vi "Pockels Cal-Process window.vi"(8 "error in (no error)":errorcluster) -> (1 "Cancelled (Left button pressed)":bool, 3 "Timed out or errored out":bool)   [LabVIEW 2017]
doc: "Use this template to create a dialog box with event handling."
uses:
  AOL Z/Typedefs/Pockels cal process refs.ctl
  <vilib>/Utility/miscctls.llb/LVPointTypeDef.ctl
  Globals/gl_Calibration globals.vi
  Global Variables/General Globals.vi
panel:
  out "error out":errorcluster
  out "Measured Power ind":dbl caption="Measured Power (mW)" min=0.0 max=10000.0 step=1.0 format="%.1f"
  out "Abort objective":bool
  out "Pockels Cal table":string[][](array[string])
  in  "Measured Power ctrl":dbl caption="Enter Measured Power (mW)" min=0.0 max=10000.0 step=1.0 format="%#_6f"
  out "Pockels cal progress bar":u8(slide) scale=0.0..100.0
  out "Next (ind)":bool
  out "Cancelled/Aborted":bool
  out "Exit":bool
  out "Abort (ind)":bool
  out "Display message":string
  in  "Cancel":bool
  in  "Next":bool
  in  "Message string":string
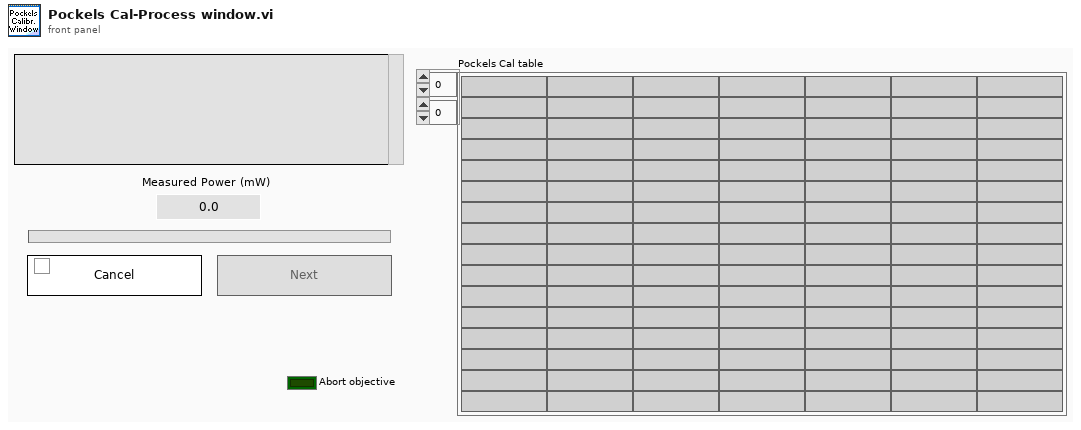
[diagram p1: front panel]
types:
  T1 = typedef "Pockels cal process refs.ctl" = cluster{"This VI":refnum<vi>, "Abort (ind)":refnum<vi>, "Next (ind)":refnum<vi>, "Cancel":refnum<vi>, "Next":refnum<vi>, "Message":refnum<vi>, "Measured Power ctrl":refnum<vi>, "Measured Power ind":refnum<vi>, "Pockels cal progress bar":refnum<vi>, "Abort this objective":refnum<vi>}
  T2 = typedef "LVPointTypeDef.ctl" = cluster{"Horizontal":i16, "Vertical":i16}
  T3 = typedef "Cal mode.ctl" = enum16{"Automatic", "Interactive"}
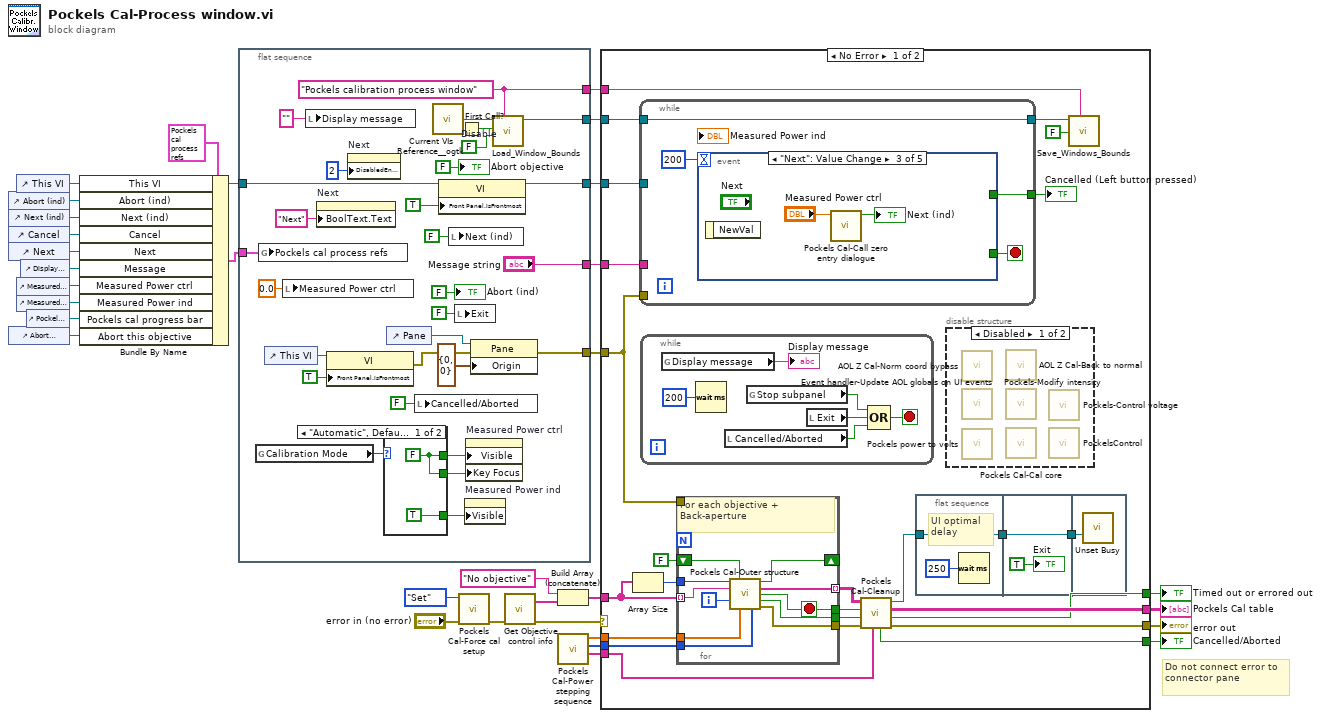
[diagram p0: block diagram]
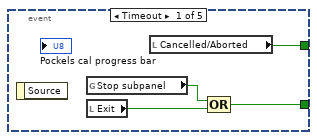
[diagram p3: hidden frame]
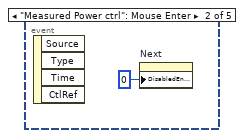
[diagram p4: hidden frame]
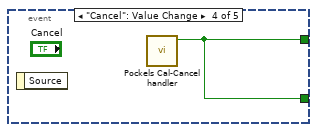
[diagram p5: hidden frame]
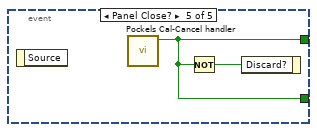
[diagram p6: hidden frame]
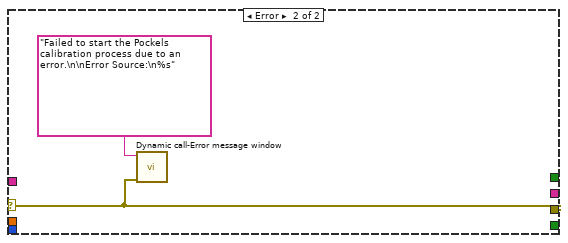
[diagram p7: hidden frame]
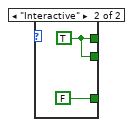
[diagram p8: hidden frame]
diagram:
  # "Do not connect error to connector pane"
  n1 = control-ref of="Abort (ind)"() -> (w26:refnum<vi>)
  n2 = control-ref of="Next (ind)"() -> (w25:refnum<vi>)
  n3 = control-ref of="Cancel"() -> (w24:refnum<vi>)
  n4 = control-ref of="Next"() -> (w23:refnum<vi>)
  n5 = control-ref of="Abort objective"() -> (w4:refnum<vi>)
  n6 = control-ref of="This VI"() -> (w22:refnum<vi>)
  n7 = control-ref of="Measured Power ctrl"() -> (w15:refnum<vi>)
  n8 = control-ref of="Measured Power ind"() -> (w1:refnum<vi>)
  n9 = control-ref of="Display message"() -> (w21:refnum<vi>)
  n10 = control-ref of="Pockels cal progress bar"() -> (w5:refnum<vi>)
  n11 = Bundle By Name(cluster=T1 {"This VI"=refnum, "Abort (ind)"=refnum, "Next (ind)"=refnum, "Cancel"=refnum, "Next"=refnum, "Message"=refnum, "Measured Power ctrl"=refnum, "Measured Power ind"=refnum, "Pockels cal progress bar"=refnum, "Abort this objective"=refnum} ("AOL Z cal wizard refs"), "This VI"=w22, "Abort (ind)"=w26, "Next (ind)"=w25, "Cancel"=w24, "Next"=w23, "Message"=w21, "Measured Power ctrl"=w15, "Measured Power ind"=w1, "Pockels cal progress bar"=w5, "Abort this objective"=w4) -> (w3:T1)
  n12 = flat-sequence {
    tunnel: ["Message string"] -> w31
    tunnel: [w58] -> w30
    tunnel: [w56] -> w27
    tunnel: [w51] -> w29
    tunnel: [w50] -> w28
    tunnel: w3 -> [w34]
    tunnel: w22 -> [w40]
    frame #0 {
      w52 = FALSE  # Disable
      w51 = "Pockels calibration process window" ("Window Name (i.e. Key)")
      n13 = global read "gl_Calibration globals.vi" "Calibration Mode"() -> (w33:T3)
      n14 = global write "gl_Calibration globals.vi" "Pockels cal process refs"(w34) -> ()
      n15 = control-ref of="This VI"() -> (w42:refnum<vi>)
      n16 = local write "Measured Power ctrl"(0.0 ("Measured Power")) -> ()
      n17 = local write "Display message"("" ("Status")) -> ()
      n18 = property on="Next" class="Bool"("BoolText.Text"="Next" ("Boolean Text.Text")) -> ()  [unwired: 2 in, 2 out]
      n19 = property on="Property Node" class="VI"(reference=w42, "Front Panel.IsFrontmost"=TRUE ("Front Panel Window:Is Frontmost")) -> (error out=w41:errorcluster)  [unwired: 1 in, 1 out]
      n20 = property on="Next" class="Bool"("DisabledEnum"=2) -> ()  [unwired: 2 in, 2 out]
      n21 = case shown="\"Automatic\", Default" w33 {
        tunnel: [w61 w63] -> w39
        tunnel: [w61 w63] -> w36
        tunnel: [TRUE FALSE] -> w32
        frame "Automatic", Default {
          w61 = FALSE
        }
        frame "Interactive" {
          w63 = TRUE
        }
      }
      n22 = control-ref of="Pane"() -> (w55:refnum<vi>)
      n23 = local write "Cancelled/Aborted"(FALSE ("Completed")) -> ()
      n24 = call <userlib>:"Current VIs Reference__ogtk.vi"() -> ("Current VI's reference"=w54:refnum<vi>)  [unwired: 5 in]
      n25 = property on="Property Node" class="VI"(reference=w40, "Front Panel.IsFrontmost"=TRUE ("Front Panel Window:Is Frontmost")) -> (reference out=w58:refnum<vi>)  [unwired: 1 in, 1 out]
      n26 = local write "Next (ind)"(FALSE ("Next (ind)")) -> ()
      n27 = local write "Exit"(FALSE ("Finished")) -> ()
      n28 = First Call?() -> (First Call?: T/F=w53:bool)
      n29 = property on="Measured Power ind" class="DigNum (strict)"("Visible"=w32) -> ()  [unwired: 2 in, 2 out]
      n30 = property on="Measured Power ctrl" class="DigNum (strict)"("Visible"=w39, "Key Focus"=w36) -> ()  [unwired: 2 in, 2 out]
      n31 = property class="Pane"(reference=w55, error in=w41, "Origin"=T2 {"Horizontal"=0, "Vertical"=0}) -> (error out=w56:errorcluster)  [unwired: 1 out]
      n32 = call "Load_Window_Bounds.vi"("Window Name (i.e. Key)"=w51, "Disable"=w52, "First Call"=w53, "Window VI's Ref"=w54) -> ("reference out"=w50:refnum<vi>)  [unwired: 4 in, 3 out]
      "Abort (ind)" <- FALSE ("Cancel ind")
      "Abort objective" <- FALSE ("Cancel ind")
    }
  }
  n33 = call "Pockels Cal-Force cal setup.vi"("error in (no error)"="error in (no error)", "Function"=enum16{"Set", "Recover"}."Set") -> ("error out"=w9:errorcluster)  [unwired: 9 in]
  n34 = call "Get Objective control info.vi"("error in (no error)"=w9) -> ("error out"=w18:errorcluster, "Objective values/strings"=w13:string[])  [unwired: 6 in, 3 out]
  n35 = Build Array (concatenate)("No objective" ("Value"), w13) -> (w12:string[])
  n36 = call "Pockels Cal-Power stepping sequence.vi"() -> ("Pockels calibration voltage steps sequence (strings)"=w17:string[], "Voltage %"=w14:u16[], "Pockels calibration voltage steps sequence"=w16:dbl[])  [unwired: 8 in, 1 out]
  n37 = case shown="No Error" w18 {
    selector: w18 -> [_ w126]
    tunnel: w31 -> [w89 _]
    tunnel: w30 -> [w88 _]
    tunnel: w29 -> [w87 _]
    tunnel: w28 -> [w85 _]
    tunnel: w27 -> [w82 _]
    tunnel: [w81 w126] -> w19
    tunnel: w12 -> [w76 _]
    tunnel: w17 -> [w69 _]
    tunnel: w16 -> [w79 _]
    tunnel: w14 -> [w78 _]
    tunnel: [w73 _] -> w7
    tunnel: [w72 _] -> w6
    tunnel: [w65 _] -> w2
    frame No Error {
      n38 = Array Size(array=w76) -> (size(s)=w77:i32)
      n39 = while {
        tunnel: w89 -> [_]
        tunnel: w82 -> [_]
        tunnel: w88 -> [_]
        tunnel: [w102] -> w74
        tunnel: w85 -> [w101]
        tunnel: [w101] -> w84
        stop <- w104 stop-if-true
        n40 = event shown="[2] \"Next\": Value Change" {
          selector: _ -> [_ _ _ _ _]
          dyn-events: _ -> [_ _ _ _ _]
          timeout: 200 -> [_ _ _ _ _]
          tunnel: [w107 _ _ w112 w114] -> w104
          tunnel: [w105 _ _ w112 w114] -> w102
          event Timeout {
            n41 = event-data() -> ()  [unwired: 1 in, 1 out]
            n42 = global read "General Globals.vi" "Stop subpanel"() -> (w106:bool)
            n43 = local read "Exit"() -> (w108:bool)
            n44 = local read "Cancelled/Aborted"() -> (w105:bool)
            n45 = Compound Arithmetic op=OR(w106, w108) -> (w107:bool)
          }
          event "Measured Power ctrl": Mouse Enter {
            n46 = event-data() -> ()  [unwired: 1 in, 4 out]
            n47 = property on="Next" class="Bool"("DisabledEnum"=0) -> ()  [unwired: 2 in, 2 out]
          }
          event "Next": Value Change {
            n48 = event-data() -> ()  [unwired: 1 in, 1 out]
            n49 = call "Pockels Cal-Call zero entry dialogue.vi"("Measured Power"="Measured Power ctrl") -> ("Next (ind)"=→"Next (ind)":bool)  [unwired: 10 in]
          }
          event "Cancel": Value Change {
            n50 = event-data() -> ()  [unwired: 1 in, 1 out]
            n51 = call "Pockels Cal-Cancel handler.vi"() -> ("Stop?"=w112:bool)  [unwired: 11 in]
          }
          event Panel Close? {
            n52 = event-data() -> ()  [unwired: 1 in, 1 out]
            n53 = call "Pockels Cal-Cancel handler.vi"() -> ("Stop?"=w114:bool)  [unwired: 11 in]
            n54 = Not(x=w114) -> (.not. x?=w113:bool)
            n55 = event-data("Discard?"=w113) -> ()  [unwired: 1 in, 1 out]
          }
        }
      }
      "Cancelled (Left button pressed)" <- w74
      n56 = while {
        stop <- w98 stop-if-true
        n57 = global read "gl_Calibration globals.vi" "Display message"() -> (→"Display message":string)
        n58 = Wait (ms)(milliseconds to wait=u32 200) -> ()  [unwired: 1 out]
        n59 = local read "Cancelled/Aborted"() -> (w95:bool)
        n60 = global read "General Globals.vi" "Stop subpanel"() -> (w100:bool)
        n61 = local read "Exit"() -> (w99:bool)
        n62 = Compound Arithmetic op=OR(w100, w99, w95) -> (w98:bool)
      }
      n63 = for {
        tunnel: [w125] -> w83 mode=indexing
        tunnel: [w115] -> w67
        tunnel: w82 -> [_]
        tunnel: [w116] -> w68
        tunnel: w77 -> [w124]
        tunnel: [w123] -> w80
        tunnel: w76 -> [w118] mode=indexing
        tunnel: w79 -> [w122]
        tunnel: w78 -> [w121]
        shift-right: [w120] -> _
        shift-left: FALSE -> [w119]
        i -> [w117]
        stop <- w115 stop-if-true
        # "For each objective + \nBack-aperture"
        n64 = call "Pockels Cal-Outer structure.vi"("Number of objectives + 1"=w124, "Skip cal for all remaining objectives?"=w119, "Objective's name"=w118, "Parent FOR loop's index"=w117, "Pockels calibration voltage steps sequence"=w122, "Voltage %"=w121) -> ("Skip cal for all remaining objectives"=w120:bool, "Results array"=w125:string[], "Cancel & Exit"=w115:bool, "Timed out or errored out"=w116:bool, "error out"=w123:errorcluster)  [unwired: 5 in]
      }
      n65 = call "Pockels Cal-Cleanup.vi"("Pockels calibration voltage steps sequence (strings)"=w69, "error in (no error)"=w80, "Timed out or error"=w68, "Cancelled/Aborted"=w67, "Calibration data (all objectives even if blank)"=w83) -> ("error out"=w81:errorcluster, "Timed out or errored out"=w72:bool, "Formatted cal table (inc. header)"=w73:string[][], "VI out"=w70:refnum<vi>, "Cancelled/Aborted"=w65:bool)  [unwired: 2 in]
      n66 = flat-sequence {
        tunnel: [w90] -> w71
        tunnel: w70 -> [w90]
        tunnel: w71 -> [w93]
        tunnel: [w93] -> w66
        tunnel: w66 -> [w94]
        frame #0 {
          # "UI optimal delay"
          n67 = Wait (ms)(milliseconds to wait=u32 250) -> ()  [unwired: 1 out]
        }
        frame #1 {
          "Exit" <- TRUE ("Finished")
        }
        frame #2 {
          n68 = call <vilib>:"Unset Busy.vi"("VI reference (current VI)"=w94) -> ()  [unwired: 10 in, 1 out]
        }
      }
      n69 = disable-structure shown="Disabled" {
        frame Disabled {
          n70 = call "AOL Z Cal-Norm coord bypass.vi"() -> ()  [unwired: 11 in, 1 out]
          n71 = call "Event handler-Update AOL globals on UI events.vi"() -> ()  [unwired: 11 in, 1 out]
          n72 = call "Pockels power to volts.vi"() -> ()  [unwired: 9 in, 3 out]
          n73 = call "AOL Z Cal-Back to normal.vi"() -> ()  [unwired: 12 in]
          n74 = call "Pockels-Modify intensity.vi"() -> ()  [unwired: 10 in, 2 out]
          n75 = call "Pockels Cal-Cal core.vi"() -> ()  [unwired: 9 in, 3 out]
          n76 = call "Pockels-Control voltage.vi"() -> ()  [unwired: 10 in, 2 out]
          n77 = call "PockelsControl.vi"() -> ()  [unwired: 11 in, 1 out]
        }
        frame Enabled {
        }
      }
      n78 = call "Save_Windows_Bounds.vi"("Window Name (i.e. Key)"=w87, "Front Panel Window:Open"=FALSE, "Window VI's Ref"=w84) -> ()  [unwired: 8 in, 1 out]
    }
    frame Error {
      n79 = call "Dynamic call-Error message window.vi"("error in (no error)"=w126, "Error Message"="Failed to start the Pockels calibration process due to an error.\n\nError Source:\n%s") -> ()  [unwired: 9 in, 1 out]
    }
  }
  "error out" <- w19
  "Pockels Cal table" <- w7
  "Timed out or errored out" <- w6
  "Cancelled/Aborted" <- w2
